vi "send_internal_trigger.vi"(7 "ensure unique insertion?":bool, 8 "error in (no error)":errorcluster, 10 "trigger":T1, 11 "ScanHeadMH100729FPGA in":refnum<class "ScanHeadMH100729FPGA.lvclass">) -> (0 "error out":errorcluster, 3 "ScanHeadMH100729FPGA out":refnum<class "ScanHeadMH100729FPGA.lvclass">)   [LabVIEW 2010, in "ScanHeadMH100729FPGA.lvclass"]
uses:
  ScanHeadMH100729FPGA.lvclass
  internal_trigger_enum.ctl
  common/classes/GenericToplevelComponent/GenericToplevelComponent/trigger_type_enum.ctl
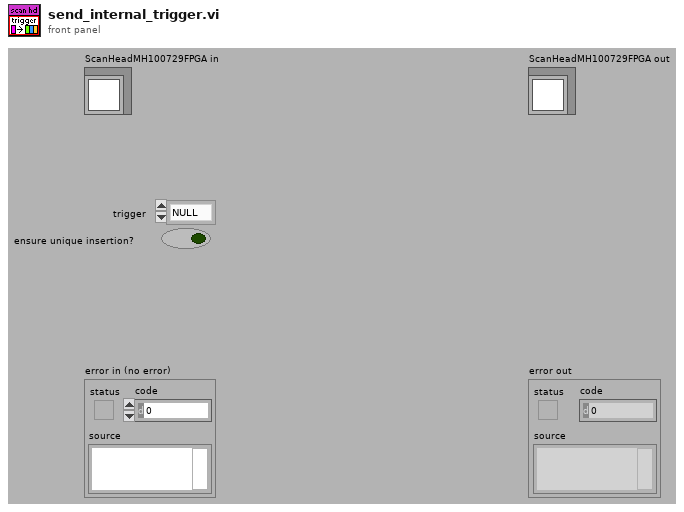
[diagram p1: front panel]
types:
  T1 = typedef "ScanHeadMH100729FPGA.lvclass/internal_trigger_enum.ctl" = enum16{"NULL", "initialise", "terminate", "start scanning", "stop scanning", "update", "fetch trajectory"}
  T2 = typedef "trigger_type_enum.ctl" = enum8{"external", "internal", "common"}
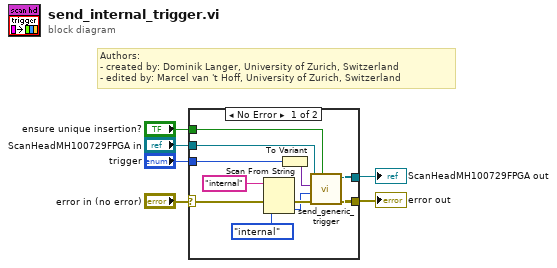
[diagram p0: block diagram]
diagram:
  # "Authors: \n- created by: Dominik Langer, University of Zurich, Switzerland\n- edited by: Marcel van 't Hoff, University of Zurich, Switzerland"
  n1 = case shown="No Error" "error in (no error)" {
    selector: "error in (no error)" -> [w11 w19]
    tunnel: [w13 w19] -> w3
    tunnel: [w12 w18] -> w5
    tunnel: "ScanHeadMH100729FPGA in" -> [w16 w18]
    tunnel: "ensure unique insertion?" -> [w15 _]
    tunnel: "trigger" -> [w17 _]
    frame No Error {
      n2 = Scan From String(input string="internal", error in=w11, default 1=trigger_type_enum."internal" ("trigger type")) -> (error out=w10:errorcluster, output 1=w9:T2)  [unwired: 2 in, 2 out]
      n3 = To Variant(anything=w17) -> (Variant=w14:variant)
      n4 = call-dynamic "send_generic_trigger.vi"("ensure unique insertion?"=w15, "error in (no error)"=w10, "trigger type"=w9, "trigger variant"=w14, "GenericToplevelComponent in"=w16) -> ("error out"=w13:errorcluster, "GenericToplevelComponent out"=w12:refnum<class "ScanHeadMH100729FPGA.lvclass">)  [unwired: 3 in, 2 out]
    }
    frame Error {
    }
  }
  "error out" <- w3
  "ScanHeadMH100729FPGA out" <- w5
